vi "Create_Object.vi"(8 "error in (no error)":errorcluster, 9 "Terminal Map in":map{string, T1}(c390), 10 "vi refnum in":refnum<vi>, 11 "Constant in":refnum<class "Constant.lvclass">) -> (0 "error out":errorcluster, 1 "Terminal Map Out":map{string, T1}(c390), 3 "Constant out":refnum<class "Constant.lvclass">)   [LabVIEW 2025, in "Constant.lvclass"]
uses:
  Constant.lvclass
  home/jake/Documents/github/LVGPT/LabVIEW/VIs/Classes/Node/Node.lvclass
  Terminal.ctl
  Node/Node.lvclass/Node.ctl
  Node/Node.lvclass
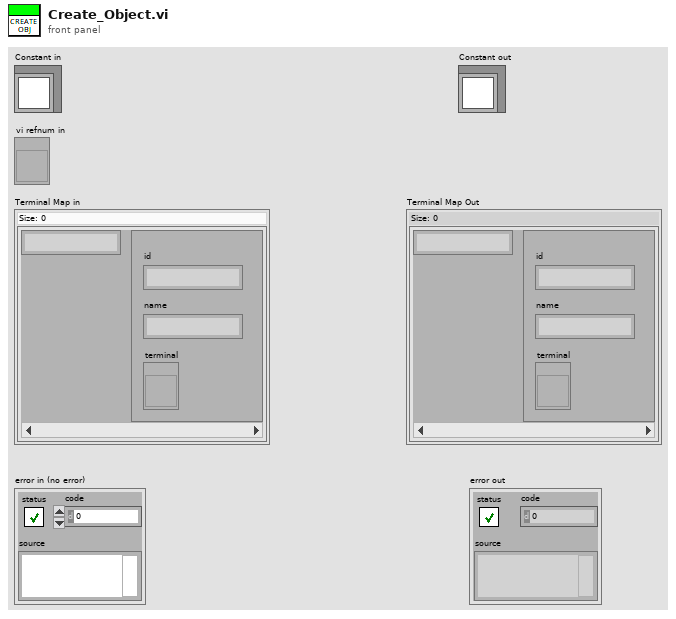
[diagram p1: front panel]
types:
  T1 = typedef "Terminal.ctl" = cluster{"id":string, "name":string, "terminal":refnum<vi>}
  T2 = typedef "LVPointTypeDef.ctl" = cluster{"Horizontal":i16, "Vertical":i16}
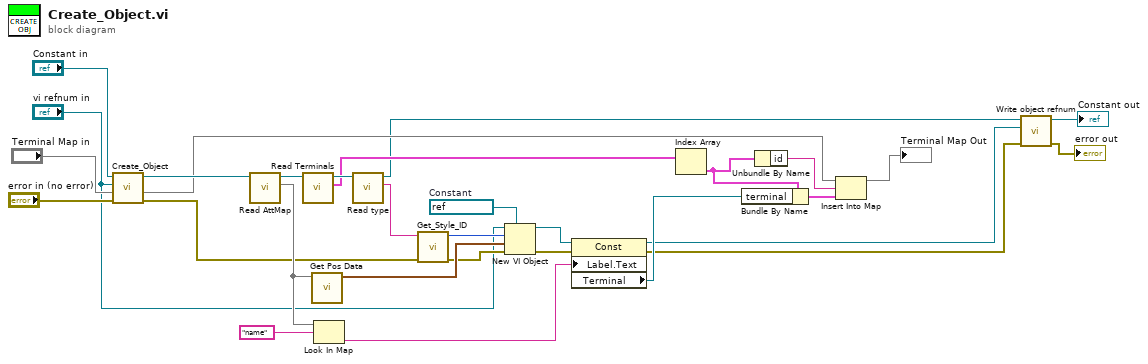
[diagram p0: block diagram]
diagram:
  w24 = refnum<vi> refnum  # Constant
  n1 = call-parent "Create_Object.vi"("error in (no error)"="error in (no error)", "Terminal Map in"="Terminal Map in", "vi refnum in"="vi refnum in", "Node in"="Constant in") -> ("error out"=w17:errorcluster, "Terminal Map Out"=w12:map{string, T1}, "Node out"=w21:refnum<class "Constant.lvclass">)  [unwired: 5 in]
  n2 = call "Read AttMap.vi"("Node in"=w21) -> ("AttMap"=w22:map{string, string}, "Node out"=w27:refnum<class "Constant.lvclass">)  [unwired: 8 in, 1 out]
  n3 = call "Read Terminals.vi"("Node in"=w27) -> ("Terminals"=w13:T1[], "Node out"=w26:refnum<class "Constant.lvclass">)  [unwired: 8 in, 1 out]
  n4 = call "Get Pos Data.vi"("AttMap"=w22) -> ("Position"=w23:T2)  [unwired: 10 in]
  n5 = Look In Map(map=w22, key="name") -> (value=w1:string)  [unwired: 1 in, 1 out]
  n6 = call "Read type.vi"("Node in"=w26) -> ("type"=w19:string, "Node out"=w7:refnum<class "Constant.lvclass">)  [unwired: 8 in, 1 out]
  n7 = call "Get_Style_ID.vi"("error in (no error)"=w17, "Style"=w19) -> ("error out"=w18:errorcluster, "style"=w20:i32)  [unwired: 7 in, 1 out]
  n8 = New VI Object(vi object class=w24, owner refnum="vi refnum in", style=w20, position/next to=w23, 8:w18) -> (object refnum=w11:refnum<vi>, 0:w10:errorcluster)  [unwired: 3 in]
  n9 = property class="Const"(reference=w11, error in=w10, "Label.Text"=w1) -> (reference out=w6:refnum<vi>, error out=w5:errorcluster, "Terminal"=w9:refnum<vi>)
  n10 = Index Array(array=w13) -> (element=w15:T1)  [unwired: 1 in]
  n11 = Bundle By Name(cluster=w15, "terminal"=w9) -> (w14:T1)
  n12 = Unbundle By Name(w15) -> ("id"=w16:string)
  n13 = Insert Into Map(map in=w12, key=w16, value=w14) -> (map out=→"Terminal Map Out":map{string, T1})  [unwired: 2 out]
  n14 = call-dynamic "Write object refnum.vi"("error in (no error)"=w5, "object refnum"=w6, "Node in"=w7) -> ("error out"=→"error out":errorcluster, "Node out"=→"Constant out":refnum<class "Constant.lvclass">)  [unwired: 7 in]
